vi "Periodic Tasks.vi"(8 "error in":errorcluster) -> ()   [LabVIEW 2012]
doc: "This VI runs in parallel to other tasks. It can contain as many user-defined periodic loops as you need. These can carry out PID or other sorts of timed response."
uses:
  <vilib>/Rock Robotics/SystemInterfaces/Utilities/FPGA_UtilitiesLED Source.ctl
  <vilib>/Rock Robotics/SystemInterfaces/Utilities/FPGA_UtilitiesLED State.ctl
  <vilib>/Rock Robotics/WPI/Joystick/WPI_JoystickGetSetRefNum.vi
  <vilib>/Rock Robotics/WPI/Solenoid/Deprecated/WPI_SolenoidSetBool.vi
  Robot Global Data.vi
  <vilib>/Rock Robotics/WPI/Compressor/WPI_CompressorGetSetRefNum.vi
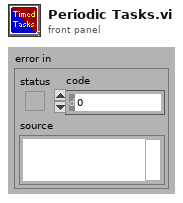
[diagram p1: front panel]
types:
  T1 = typedef "FPGA_UtilitiesLED State.ctl" = enum16{"Off", "On", "Toggle"}
  T2 = typedef "FPGA_UtilitiesLED Source.ctl" = enum16{"User LED", "FPGA LED"}
  T3 = typedef "WPI_JoystickDevRef.ctl" = cluster{"Device":T4}
  T4 = typedef "WPI_JoystickDeviceEnum.ctl" = enum16{"USB 1", "USB 2", "USB 3", "USB 4", "Kinect 1", "Kinect 2"}
  T5 = typedef "WPI_JoystickButtonState.ctl" = cluster{"Button 1":bool, "Button 2":bool, "Button 3":bool, "Button 4":bool, "Button 5":bool, "Button 6":bool, "Button 7":bool, "Button 8":bool, "Button 9":bool, "Button 10":bool, "Button 11":bool, "Button 12":bool}
  T6 = typedef "WPI_SolenoidDevRef.ctl" = cluster{"DevStatus":errorcluster, "Solenoid Module":T7, "Forward Solenoid Channel":T8, "Reverse Solenoid Channel":T8}
  T7 = typedef "FPGA_TypedefSolenoidModule.ctl" = enum16{"Solenoid Module 1", "Solenoid Module 2"}
  T8 = typedef "WPI_SolenoidChannel.ctl" = enum8{"Solenoid 1", "Solenoid 2", "Solenoid 3", "Solenoid 4", "Solenoid 5", "Solenoid 6", "Solenoid 7", "Solenoid 8", "Invalid"}
  T9 = typedef "WPI_CompressorDevRef.ctl" = cluster{"DevStatus":errorcluster, "DigitalInputDevRef":T10, "RelayDevRef":T13}
  T10 = typedef "WPI_DigitalInputDevRef.ctl" = cluster{"DevStatus":errorcluster, "DIO Channel":T11, "Digital Module":T12}
  T11 = typedef "FPGA_DIOChannel.ctl" = enum8{"DIO 1", "DIO 2", "DIO 3", "DIO 4", "DIO 5", "DIO 6", "DIO 7", "DIO 8", "DIO 9", "DIO 10", "DIO 11", "DIO 12", "DIO 13", "DIO 14", "Invalid"}
  T12 = typedef "FPGA_TypedefDigitalModule.ctl" = enum16{"Digital Module 1", "Digital Module 2"}
  T13 = typedef "WPI_RelayDevRef.ctl" = cluster{"DevStatus":errorcluster, "Relay Channel":T14, "Digital Module":T12, "Relay Direction":T15}
  T14 = typedef "FPGA_DIORelayChannel.ctl" = enum8{"Relay 1", "Relay 2", "Relay 3", "Relay 4", "Relay 5", "Relay 6", "Relay 7", "Relay 8", "Invalid"}
  T15 = typedef "WPI_RelayDirection.ctl" = enum16{"Both directions", "Forward only", "Reverse only"}
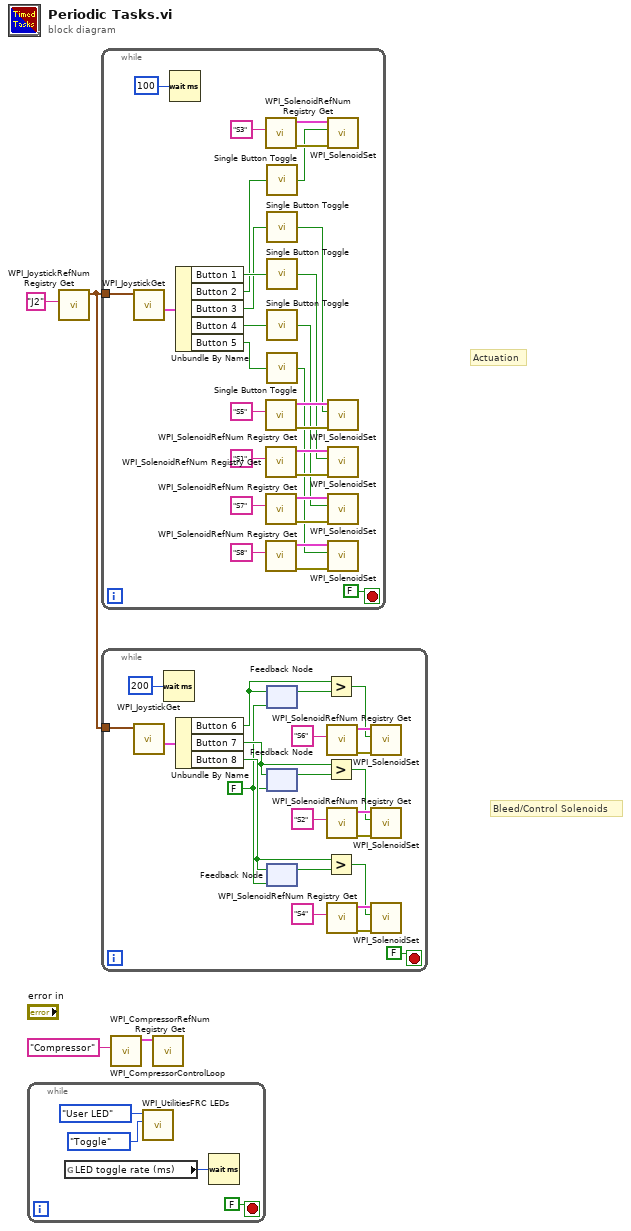
[diagram p0: block diagram]
diagram:
  # "Actuation"
  # "Bleed/Control Solenoids"
  n1 = while {
    stop <- FALSE stop-if-true
    n2 = global read "Robot Global Data.vi" "LED toggle rate (ms)"() -> (w5:u32)
    n3 = call <vilib>:"WPI_UtilitiesFRC LEDs.vi"("State"=FPGA_UtilitiesLED_State."Toggle", "LED Type"=FPGA_UtilitiesLED_Source."User LED") -> ()  [unwired: 1 in, 9 out]
    n4 = Wait (ms)(milliseconds to wait=w5) -> ()  [unwired: 1 out]
  }
  n5 = call <vilib>:"WPI_JoystickRefNum Registry Get.vi"("refnum name"="J2") -> ("JoystickDevRef"=w1:T3)  [unwired: 1 in, 9 out]
  n6 = while {
    tunnel: w1 -> [w15]
    stop <- FALSE stop-if-true
    n7 = call <vilib>:"WPI_JoystickGet.vi"("JoystickDevRef"=w15) -> ("Buttons"=w14:T5)  [unwired: 1 in, 5 out]
    n8 = Wait (ms)(milliseconds to wait=u32 100) -> ()  [unwired: 1 out]
    n9 = Unbundle By Name(w14) -> ("Button 1"=w13:bool, "Button 2"=w12:bool, "Button 3"=w11:bool, "Button 4"=w10:bool, "Button 5"=w9:bool)
    n10 = call <vilib>:"WPI_SolenoidRefNum Registry Get.vi"("refnum name"="S3") -> ("error out"=w32:errorcluster, "SolenoidDevRef"=w31:T6)  [unwired: 9 in]
    n11 = call <vilib>:"WPI_SolenoidRefNum Registry Get.vi"("refnum name"="S5") -> ("error out"=w29:errorcluster, "SolenoidDevRef"=w28:T6)  [unwired: 9 in]
    n12 = call <vilib>:"WPI_SolenoidRefNum Registry Get.vi"("refnum name"="S1") -> ("error out"=w35:errorcluster, "SolenoidDevRef"=w34:T6)  [unwired: 9 in]
    n13 = call <vilib>:"WPI_SolenoidRefNum Registry Get.vi"("refnum name"="S7") -> ("error out"=w26:errorcluster, "SolenoidDevRef"=w25:T6)  [unwired: 9 in]
    n14 = call <vilib>:"WPI_SolenoidRefNum Registry Get.vi"("refnum name"="S8") -> ("error out"=w23:errorcluster, "SolenoidDevRef"=w22:T6)  [unwired: 9 in]
    n15 = call "Single Button Toggle.vi"("Input"=w12) -> ("Output"=w16:bool)
    n16 = call "Single Button Toggle.vi"("Input"=w11) -> ("Output"=w17:bool)
    n17 = call "Single Button Toggle.vi"("Input"=w13) -> ("Output"=w20:bool)
    n18 = call "Single Button Toggle.vi"("Input"=w10) -> ("Output"=w18:bool)
    n19 = call "Single Button Toggle.vi"("Input"=w9) -> ("Output"=w19:bool)
    n20 = call-poly <vilib>:"WPI_SolenoidSet.vi"("error in (no error)"=w32, "Value"=w16, "SolenoidDevRef"=w31) -> ()  [unwired: 7 in, 2 out]
    n21 = call-poly <vilib>:"WPI_SolenoidSet.vi"("error in (no error)"=w29, "Value"=w17, "SolenoidDevRef"=w28) -> ()  [unwired: 7 in, 2 out]
    n22 = call-poly <vilib>:"WPI_SolenoidSet.vi"("error in (no error)"=w35, "Value"=w20, "SolenoidDevRef"=w34) -> ()  [unwired: 7 in, 2 out]
    n23 = call-poly <vilib>:"WPI_SolenoidSet.vi"("error in (no error)"=w26, "Value"=w18, "SolenoidDevRef"=w25) -> ()  [unwired: 7 in, 2 out]
    n24 = call-poly <vilib>:"WPI_SolenoidSet.vi"("error in (no error)"=w23, "Value"=w19, "SolenoidDevRef"=w22) -> ()  [unwired: 7 in, 2 out]
  }
  n25 = while {
    tunnel: w1 -> [w38]
    stop <- FALSE stop-if-true
    w42 = FALSE
    n26 = call <vilib>:"WPI_JoystickGet.vi"("JoystickDevRef"=w38) -> ("Buttons"=w60:T5)  [unwired: 1 in, 5 out]
    n27 = Wait (ms)(milliseconds to wait=u32 200 ("millisecond multiple")) -> ()  [unwired: 1 out]
    n28 = Unbundle By Name(w60) -> ("Button 6"=w45:bool, "Button 7"=w56:bool, "Button 8"=w43:bool)
    n29 = feedback #1(w42) -> (w46:bool)
    n30 = feedback-in #1(w45) -> ()
    n31 = feedback #2(w42) -> (w55:bool)
    n32 = feedback-in #2(w56) -> ()
    n33 = feedback #3(w42) -> (w44:bool)
    n34 = feedback-in #3(w43) -> ()
    n35 = Greater?(x=w45, y=w46) -> (0:w40:bool)
    n36 = Greater?(x=w56, y=w55) -> (0:w53:bool)
    n37 = Greater?(x=w43, y=w44) -> (0:w41:bool)
    n38 = call <vilib>:"WPI_SolenoidRefNum Registry Get.vi"("refnum name"="S6") -> ("error out"=w49:errorcluster, "SolenoidDevRef"=w48:T6)  [unwired: 9 in]
    n39 = call <vilib>:"WPI_SolenoidRefNum Registry Get.vi"("refnum name"="S2") -> ("error out"=w59:errorcluster, "SolenoidDevRef"=w58:T6)  [unwired: 9 in]
    n40 = call <vilib>:"WPI_SolenoidRefNum Registry Get.vi"("refnum name"="S4") -> ("error out"=w52:errorcluster, "SolenoidDevRef"=w51:T6)  [unwired: 9 in]
    n41 = call-poly <vilib>:"WPI_SolenoidSet.vi"("error in (no error)"=w49, "Value"=w40, "SolenoidDevRef"=w48) -> ()  [unwired: 7 in, 2 out]
    n42 = call-poly <vilib>:"WPI_SolenoidSet.vi"("error in (no error)"=w59, "Value"=w53, "SolenoidDevRef"=w58) -> ()  [unwired: 7 in, 2 out]
    n43 = call-poly <vilib>:"WPI_SolenoidSet.vi"("error in (no error)"=w52, "Value"=w41, "SolenoidDevRef"=w51) -> ()  [unwired: 7 in, 2 out]
  }
  n44 = call <vilib>:"WPI_CompressorRefNum Registry Get.vi"("refnum name"="Compressor") -> ("CompressorDevRef"=w4:T9)  [unwired: 9 in, 1 out]
  n45 = call <vilib>:"WPI_CompressorControlLoop.vi"("CompressorDevRef"=w4) -> ()  [unwired: 11 in]
